vi "Get Team List from XML.vi"(11 "XML In":string) -> (3 "Team List Array":T1)   [LabVIEW 2013]
uses:
  Team_List_Array_Ctrl.ctl
  Team_List_Ctrl.ctl
  <vilib>/xml/Close Reference(Node).vi
  <vilib>/xml/NI_XML.lvlib
  <resource>/objmgr/DOMUserDefRef.rc
panel:
  out "error out":errorcluster
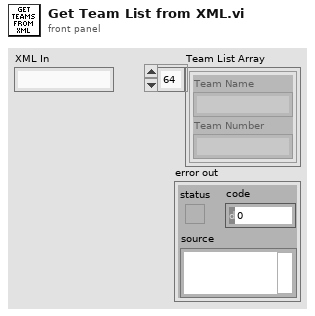
[diagram p1: front panel]
types:
  T1 = typedef "Team_List_Array_Ctrl.ctl" = T2[]
  T2 = typedef "Team_List_Ctrl.ctl" = cluster{"Team Name":string, "Team Number":string}
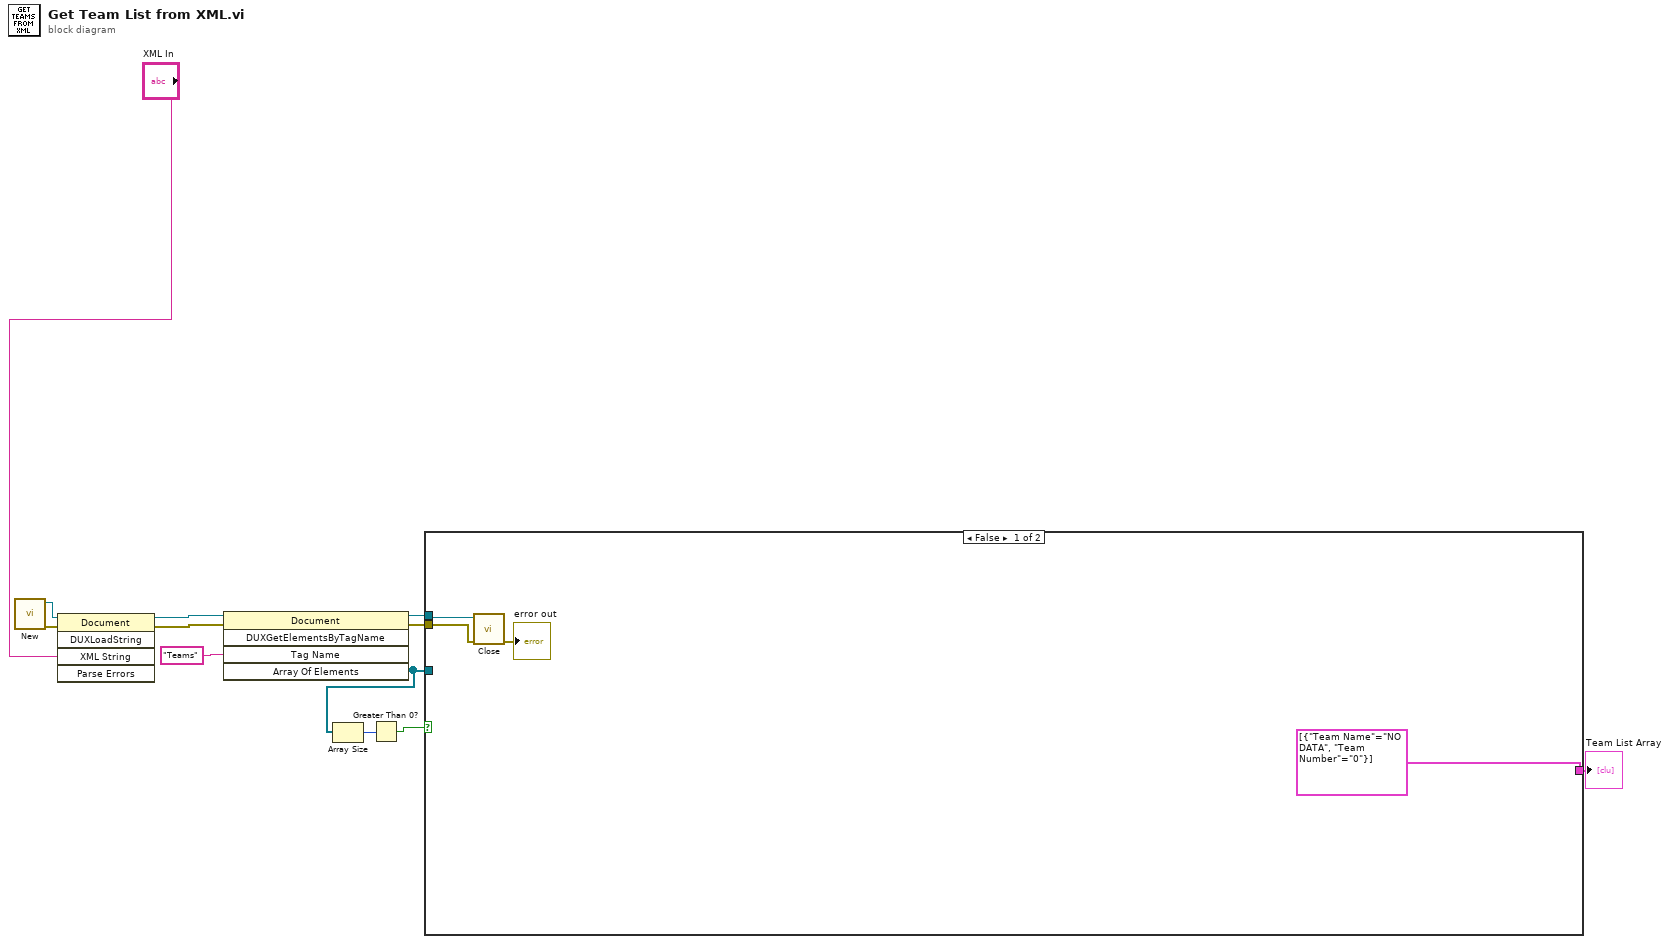
[diagram p0: block diagram]
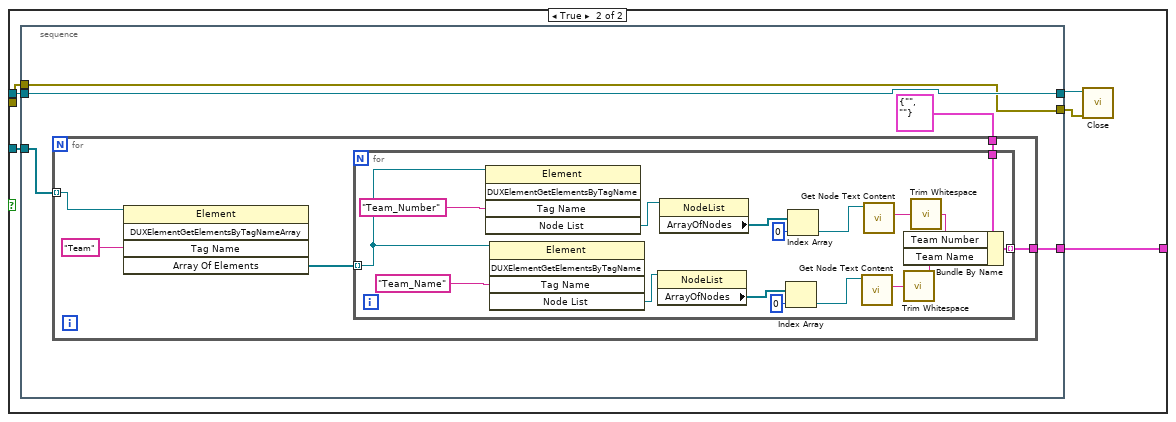
[diagram p2: hidden frame]
diagram:
  n1 = call <vilib>:"New.vi"() -> ("error out"=w9:errorcluster, "DOM document out"=w6:refnum<k20>)  [unwired: 8 in]
  n2 = invoke class="Document" method="DUXLoadString"(reference=w6, error in=w9, "XML String"="XML In") -> (reference out=w7:refnum<k20>, error out=w8:errorcluster)  [unwired: 2 in, 3 out]
  n3 = invoke class="Document" method="DUXGetElementsByTagName"(reference=w7, error in=w8, "Tag Name"="Teams") -> (reference out=w10:refnum<k20>, error out=w11:errorcluster, "Array Of Elements"=w1:refnum<k20>[])  [unwired: 2 in, 2 out]
  n4 = Array Size(array=w1) -> (size(s)=w3:i32)
  n5 = Greater Than 0?(x=w3) -> (x > 0?=w2:bool)
  n6 = case shown="False" w2 {
    tunnel: [T2[] [{"Team Name"="NO DATA", "Team Number"="0"}] w22] -> w12
    tunnel: w11 -> [w15 w19]
    tunnel: w10 -> [w16 w18]
    tunnel: w1 -> [_ w17]
    frame False {
      n7 = call-poly <vilib>:"Close.vi"("error in (no error)"=w15, "node"=w16) -> ("error out"=→"error out":errorcluster)  [unwired: 7 in]
    }
    frame True {
      n8 = stacked-sequence {
        tunnel: w17 -> [w27]
        tunnel: w18 -> [w25]
        tunnel: [w25] -> w21
        tunnel: [w24] -> w20
        tunnel: w19 -> [w24]
        tunnel: [w23] -> w22
        frame #0 {
          n9 = for {
            tunnel: w27 -> [w31] mode=indexing
            tunnel: T2 {"Team Name"="", "Team Number"=""} -> [w29]
            tunnel: [w28] -> w23
            n10 = invoke class="Element" method="DUXElementGetElementsByTagNameArray"(reference=w31, "Tag Name"="Team") -> ("Array Of Elements"=w30:refnum<k20>[])  [unwired: 3 in, 4 out]
            n11 = for {
              tunnel: w30 -> [w47] mode=indexing
              tunnel: w29 -> [w38]
              tunnel: [w35] -> w28 mode=indexing
              n12 = invoke class="Element" method="DUXElementGetElementsByTagName"(reference=w47, "Tag Name"="Team_Number") -> ("Node List"=w39:refnum<k20>)  [unwired: 3 in, 4 out]
              n13 = invoke class="Element" method="DUXElementGetElementsByTagName"(reference=w47, "Tag Name"="Team_Name") -> ("Node List"=w46:refnum<k20>)  [unwired: 3 in, 4 out]
              n14 = property class="NodeList"(reference=w46) -> ("ArrayOfNodes"=w45:refnum<k20>[])  [unwired: 1 in, 2 out]
              n15 = property class="NodeList"(reference=w39) -> ("ArrayOfNodes"=w40:refnum<k20>[])  [unwired: 1 in, 2 out]
              n16 = Index Array(array=w45, index=0) -> (element=w43:refnum<k20>)
              n17 = Index Array(array=w40, index=0) -> (element=w42:refnum<k20>)
              n18 = call <vilib>:"Get Node Text Content.vi"("node in"=w43) -> ("node text"=w36:string)  [unwired: 8 in, 2 out]
              n19 = call <vilib>:"Get Node Text Content.vi"("node in"=w42) -> ("node text"=w37:string)  [unwired: 8 in, 2 out]
              n20 = call <vilib>:"Trim Whitespace.vi"("string"=w36) -> ("trimmed string"=w33:string)  [unwired: 1 in]
              n21 = call <vilib>:"Trim Whitespace.vi"("string"=w37) -> ("trimmed string"=w34:string)  [unwired: 1 in]
              n22 = Bundle By Name(cluster=w38, "Team Number"=w34, "Team Name"=w33) -> (w35:T2)
            }
          }
        }
      }
      n23 = call-poly <vilib>:"Close.vi"("error in (no error)"=w20, "node"=w21) -> ()  [unwired: 7 in, 1 out]
    }
  }
  "Team List Array" <- w12
